vi "Read Profibus Baud rate.vi"(8 "error in (no error)":errorcluster, 11 "Profibus in":refnum<class "Profibus.lvclass">) -> (0 "error out":errorcluster, 2 "Profibus Baud rate":i32(listbox)=6, 3 "Profibus out":refnum<class "Profibus.lvclass">)   [LabVIEW 2016, in "Profibus.lvclass"]
uses:
  Profibus.lvclass
  Profibus.lvclass/Profibus.ctl
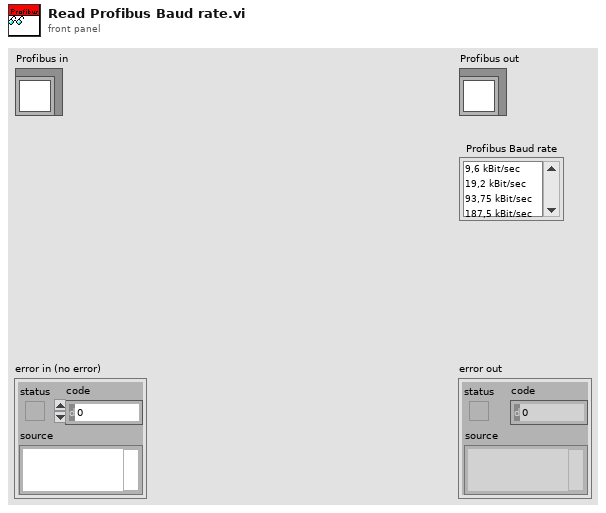
[diagram p1: front panel]
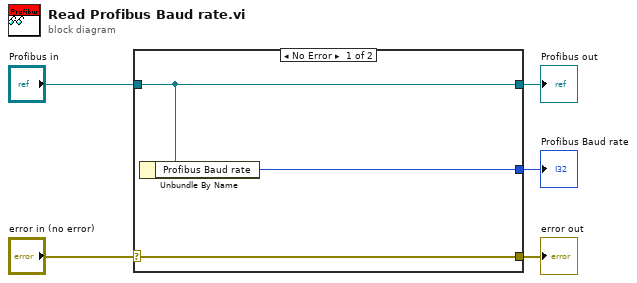
[diagram p0: block diagram]
diagram:
  n1 = case shown="No Error" "error in (no error)" {
    selector: "error in (no error)" -> [w8 w9]
    tunnel: [w8 w9] -> w4
    tunnel: [w7 w10] -> w2
    tunnel: "Profibus in" -> [w7 w10]
    tunnel: [w6 _] -> w1
    frame No Error {
      n2 = Unbundle By Name(w7) -> ("Profibus Baud rate"=w6:i32)
    }
    frame Error {
    }
  }
  "error out" <- w4
  "Profibus out" <- w2
  "Profibus Baud rate" <- w1
